vi "WriteFifos.vi"(4 "EnableGalvoDataStream":bool, 6 "EnableRawDataStream":bool, 8 "AcqStatusOut":T1, 9 "FrameTagDataPack":u64, 10 "GalvoDataPack":u64[](array[numeric])=[0, 0], 11 "PmtDataPack":u64) -> (0 "FrameTagFifoTimeouts":u64, 1 "ShortPmtDataFifoTimeouts":u64, 2 "GalvoDataFifoTimeouts":u64, 3 "PmtDataFifoTimeouts":u64)   [LabVIEW 2015]
uses:
  Typedefs/AcqStatus.ctl
  <vilib>/rvi/interface/RandomDataEmulation/niFpgaRandomDataHandleErrors.vi
  <vilib>/rvi/interface/RandomDataEmulation/nirviRandomDataMultiElementFPGAFIFO.vi
  <instcachedir>/0/nirviRandomDataMultiElementFPGAFIFO_8F99493546E24284B0D6A8E519C457F7.lvgen/nirviRandomDataMultiElementFPGAFIFO_8F99493546E24284B0D6A8E519C457F7_000.vi
  <vilib>/rvi/DataTransferAndStorage/Container/XNode/niFpgaContainer.xnode
  <vilib>/rvi/interface/RandomDataEmulation/nirviRandomDataFpgaReadWriteTemplate.vi
  <vilib>/rvi/interface/RandomDataEmulation/nirviRandomDataFpgaMultiElementTemplate.vi
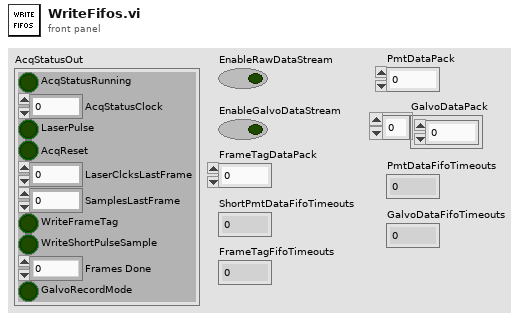
[diagram p1: front panel]
types:
  T1 = typedef "AcqStatus.ctl" = cluster{"AcqStatusRunning":bool, "AcqStatusClock":u64, "LaserPulse":bool, "AcqReset":bool, "LaserClcksLastFrame":u32, "SamplesLastFrame":u32, "WriteFrameTag":bool, "WriteShortPulseSample":bool, "Frames Done":u32, "GalvoRecordMode":bool}
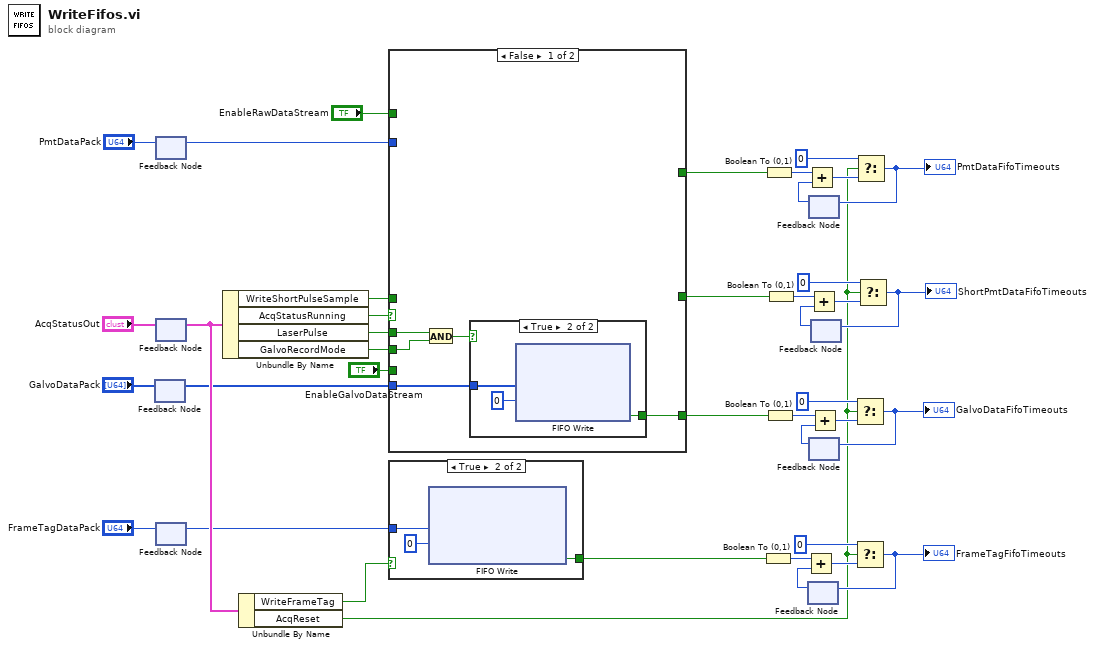
[diagram p0: block diagram]
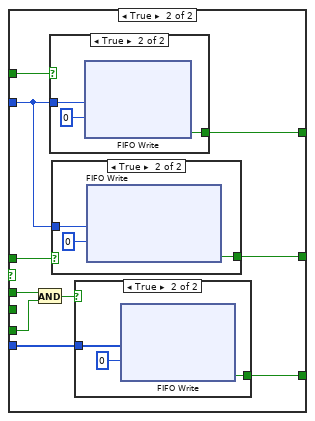
[diagram p4: hidden frame]
diagram:
  n1 = feedback-in #1("GalvoDataPack") -> ()
  n2 = feedback #1() -> (w23:u64[])  [unwired: 1 in]
  n3 = feedback-in #2("PmtDataPack") -> ()
  n4 = feedback #2() -> (w22:u64)  [unwired: 1 in]
  n5 = feedback-in #3("AcqStatusOut") -> ()
  n6 = feedback #3() -> (w24:T1)  [unwired: 1 in]
  n7 = feedback-in #4("FrameTagDataPack") -> ()
  n8 = feedback #4() -> (w3:u64)  [unwired: 1 in]
  n9 = Unbundle By Name(w24) -> ("WriteShortPulseSample"=w19:bool, "AcqStatusRunning"=w38:bool, "LaserPulse"=w39:bool, "GalvoRecordMode"=w2:bool)
  n10 = Unbundle By Name(w24) -> ("WriteFrameTag"=w18:bool, "AcqReset"=w5:bool)
  n11 = case shown="False" w38 {
    tunnel: w22 -> [_ w50]
    tunnel: w23 -> [w42 w58]
    tunnel: w39 -> [w44 w55]
    tunnel: [w41 w57] -> w37
    tunnel: [_ w56] -> w36
    tunnel: "EnableGalvoDataStream" -> [_ w54]
    tunnel: "EnableRawDataStream" -> [_ w52]
    tunnel: w19 -> [_ w51]
    tunnel: [_ w49] -> w7
    tunnel: w2 -> [w43 _]
    frame False {
      n12 = And(x=w44, y=w43) -> (x .and. y?=w45:bool)
      n13 = case shown="True" w45 {
        tunnel: w42 -> [_ w47]
        tunnel: [_ w46] -> w41
        frame False {
        }
        frame True {
          n14 = xnode ("FIFO Write")("Element"=w47, "Timeout"=0) -> ("Timed Out?"=w46:bool)  [unwired: 1 in, 1 out]
        }
      }
    }
    frame True {
      n15 = And(x=w55, y=w54) -> (x .and. y?=w53:bool)
      n16 = case shown="True" w52 {
        tunnel: w50 -> [_ w63]
        tunnel: [_ w62] -> w56
        frame False {
        }
        frame True {
          n17 = xnode ("FIFO Write")("Element"=w63, "Timeout"=0) -> ("Timed Out?"=w62:bool)  [unwired: 1 in, 1 out]
        }
      }
      n18 = case shown="True" w51 {
        tunnel: w50 -> [_ w60]
        tunnel: [_ w59] -> w49
        frame False {
        }
        frame True {
          n19 = xnode ("FIFO Write")("Element"=w60, "Timeout"=0) -> ("Timed Out?"=w59:bool)  [unwired: 1 in, 1 out]
        }
      }
      n20 = case shown="True" w53 {
        tunnel: w58 -> [_ w66]
        tunnel: [_ w65] -> w57
        frame False {
        }
        frame True {
          n21 = xnode ("FIFO Write")("Element"=w66, "Timeout"=0) -> ("Timed Out?"=w65:bool)  [unwired: 1 in, 1 out]
        }
      }
    }
  }
  n22 = case shown="True" w18 {
    tunnel: w3 -> [_ w69]
    tunnel: [_ w68] -> w6
    frame False {
    }
    frame True {
      n23 = xnode ("FIFO Write")("Element"=w69, "Timeout"=0) -> ("Timed Out?"=w68:bool)  [unwired: 1 in, 1 out]
    }
  }
  n24 = Boolean To (0,1)(Boolean=w6) -> (0, 1=w12:i16)
  n25 = Boolean To (0,1)(Boolean=w36) -> (0, 1=w35:i16)
  n26 = Boolean To (0,1)(Boolean=w37) -> (0, 1=w25:i16)
  n27 = Boolean To (0,1)(Boolean=w7) -> (0, 1=w13:i16)
  n28 = feedback #5() -> (w11:u64)  [unwired: 1 in]
  n29 = Add(x=w12, y=w11) -> (x+y=w10:u64)
  n30 = feedback #6() -> (w33:u64)  [unwired: 1 in]
  n31 = Add(x=w35, y=w33) -> (x+y=w32:u64)
  n32 = feedback #7() -> (w26:u64)  [unwired: 1 in]
  n33 = Add(x=w25, y=w26) -> (x+y=w27:u64)
  n34 = feedback #8() -> (w14:u64)  [unwired: 1 in]
  n35 = Add(x=w13, y=w14) -> (x+y=w15:u64)
  n36 = Select(t=u64 0, s=w5, f=w27) -> (s? t:f=w28:u64)
  "GalvoDataFifoTimeouts" <- w28
  n37 = feedback-in #7(w28) -> ()
  n38 = Select(t=u64 0, s=w5, f=w10) -> (s? t:f=w9:u64)
  "FrameTagFifoTimeouts" <- w9
  n39 = feedback-in #5(w9) -> ()
  n40 = Select(t=u64 0, s=w5, f=w32) -> (s? t:f=w31:u64)
  "PmtDataFifoTimeouts" <- w31
  n41 = feedback-in #6(w31) -> ()
  n42 = Select(t=u64 0, s=w5, f=w15) -> (s? t:f=w16:u64)
  "ShortPmtDataFifoTimeouts" <- w16
  n43 = feedback-in #8(w16) -> ()
